vi "PeriodicTaskSevenSegment.vi"(8 "Error In":errorcluster, 9 "Smart Write? (T)":bool=TRUE, 10 "Value To Display":u16, 11 "LINX Resource":T1) -> (0 "Error Out":errorcluster, 2 "Response":u8[](array[numeric]), 3 "LINX Resource":T1)   [LabVIEW 2020, in "LMH-LINX.lvlib" / "Interaction Parts Kit.lvlib"]
doc: "Updates the integer displayed on the 7 segment display"
uses:
  Interaction Parts Kit.lvlib
  Private/Type Defs/LINX Ref.ctl
  Private/Type Defs/Platform.ctl
  Private/Type Defs/Interface.ctl
  Private/Device/Type Defs/LINX Device Config.ctl
  Private/Device/Type Defs/TCP Config.ctl
  Private/Device/Type Defs/Channels.ctl
  LMH-LINX.lvlib
  Private/Device/Device.lvlib
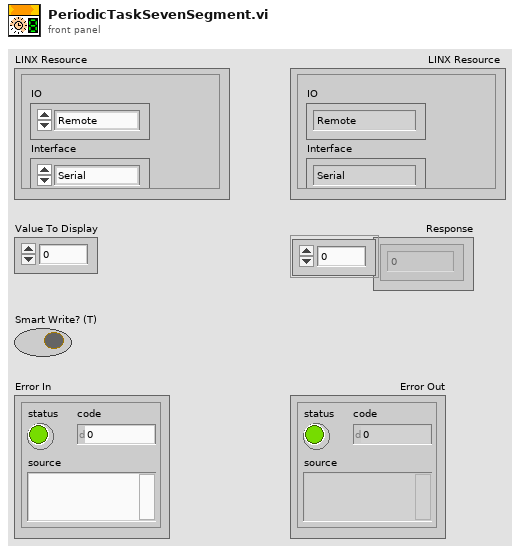
[diagram p1: front panel]
types:
  T1 = typedef "LMH-LINX.lvlib/LINX Ref.ctl" = cluster{"IO":T2, "Interface":T3, "LINX Device Config":T4}
  T2 = typedef "LMH-LINX.lvlib/Platform.ctl" = enum16{"Remote", "Local"}
  T3 = typedef "LMH-LINX.lvlib/Interface.ctl" = enum16{"Serial", "TCP"}
  T4 = typedef "LMH-LINX.lvlib/Device.lvlib/LINX Device Config.ctl" = cluster{"Interface":T3, "COM Port":refnum<visa-resource-name>, "TCP Configuration":T5, "Device Family":u8, "Device ID":u8, "Device Name":string, "TCP Ref":refnum<k5>, "Channels":T6}
  T5 = typedef "LMH-LINX.lvlib/Device.lvlib/TCP Config.ctl" = cluster{"IP Address":string, "Port":u16}
  T6 = typedef "LMH-LINX.lvlib/Channels.ctl" = cluster{"DI":u8[], "DO":u8[], "AI":u8[], "AO":u8[], "PWM":u8[], "QE":u8[], "UART":u8[], "I2C 2":u8[], "SPI":u8[], "CAN":u8[], "Servo":u8[], "AI Ref (V)":dbl, "AI Resolution (Bits)":u8, "AO Ref (V)":dbl, "AO Resolution (Bits)":u8}
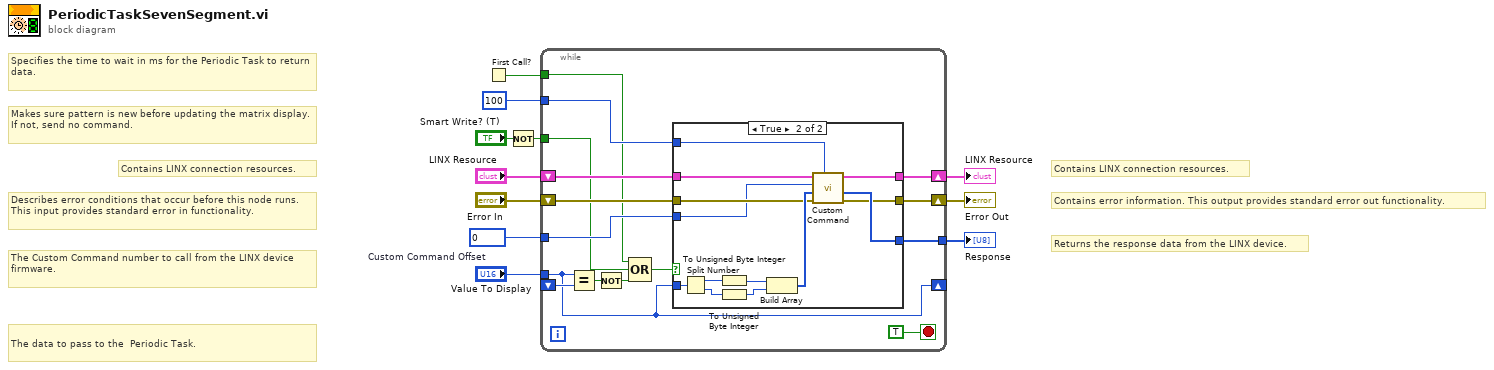
[diagram p0: block diagram]
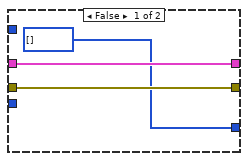
[diagram p2: hidden frame]
diagram:
  w5 = u16 0  # Custom Command Offset
  # "Makes sure pattern is new before updating the matrix display.  If not, send no command."
  # "The data to pass to the  Periodic Task."
  # "Specifies the time to wait in ms for the Periodic Task to return data."
  # "The Custom Command number to call from the LINX device firmware."
  # "Returns the response data from the LINX device."
  # "Contains LINX connection resources."
  # "Contains error information. This output provides standard error out functionality."
  # "Contains LINX connection resources."
  # "Describes error conditions that occur before this node runs. This input provides standard error in functionality."
  n1 = First Call?() -> (First Call?: T/F=w1:bool)
  n2 = Not(x="Smart Write? (T)") -> (.not. x?=w2:bool)
  n3 = while {
    tunnel: [w22] -> w7
    tunnel: 100 ("Timeout (100 ms)") -> [w21]
    tunnel: w5 -> [w20]
    shift-right: [w23] -> w8
    shift-left: "LINX Resource" -> [w26]
    shift-right: [w24] -> w9
    shift-left: "Error In" -> [w25]
    shift-right: [w16] -> _
    shift-left: _ -> [w18]
    tunnel: "Value To Display" -> [w16]
    tunnel: w2 -> [w13]
    tunnel: w1 -> [w12]
    stop <- TRUE stop-if-true
    n4 = Equal?(x=w16, y=w18) -> (x = y?=w17:bool)
    n5 = Not(x=w17) -> (.not. x?=w15:bool)
    n6 = Compound Arithmetic op=OR(w12, w13, w15) -> (w14:bool)
    n7 = case shown="True" w14 {
      tunnel: w26 -> [w29 w36]
      tunnel: w25 -> [w28 w32]
      tunnel: [w28 w33] -> w24
      tunnel: [w29 w35] -> w23
      tunnel: [u8[] [] ("Response") w34] -> w22
      tunnel: w21 -> [_ w30]
      tunnel: w20 -> [_ w31]
      tunnel: w16 -> [_ w42]
      frame False {
      }
      frame True {
        n8 = Split Number(x=w42) -> (hi(x)=w41:u8, lo(x)=w40:u8)
        n9 = To Unsigned Byte Integer(number=w41) -> (unsigned 8bit integer=w38:u8)
        n10 = To Unsigned Byte Integer(number=w40) -> (unsigned 8bit integer=w39:u8)
        n11 = Build Array(w38, w39) -> (w37:u8[])
        n12 = call "Custom Command.vi"("Timeout (100 ms)"=w30, "Error In"=w32, "Data"=w37, "Custom Command Number"=w31, "LINX Resource"=w36) -> ("Error Out"=w33:errorcluster, "Response"=w34:u8[], "LINX Resource"=w35:T1)  [unwired: 3 in, 1 out]
      }
    }
  }
  "Error Out" <- w9
  "LINX Resource" <- w8
  "Response" <- w7
